vi "Actor Core.vi"(8 "error in":errorcluster, 11 "TestQList in":refnum<class "TestQList.lvclass">) -> (0 "error out":errorcluster, 3 "Actor out":refnum<class "Actor.lvclass">)   [LabVIEW 2019, in "TestQList.lvclass"]
doc: "(<B>Filename</B>: Actor Framework.lvlib:Actor.lvclass:Actor Core.vi)\n\nReceives messages to the actor, reacts to them, and initiates any error handling that may shut the actor down.\n\nDescendant classes may override this VI to append parallel tasks for the actor to complete while it handles messages. Overrides use the Call Parent Method node."
uses:
  TestQList.lvclass
  C:/Program Files/National Instruments/LabVIEW 2019/vi.lib/ActorFramework/Actor/Actor.lvclass
  <vilib>/ActorFramework/Actor/Actor.lvclass
  Queued Listbox.xctl
  <vilib>/ActorFramework/Actor/Actor.lvclass/Actor.ctl
  <vilib>/ActorFramework/Message Enqueuer/Message Enqueuer.lvclass/Message Enqueuer.ctl
  <vilib>/ActorFramework/Message Enqueuer/Init from Existing Queue.vi
  <vilib>/ActorFramework/Message Enqueuer/Enqueue.vi
  <vilib>/ActorFramework/Stop Msg/Stop Msg.lvclass
  C:/Program Files/National Instruments/LabVIEW 2019/vi.lib/ActorFramework/Message/Message.lvclass
  <vilib>/ActorFramework/Message Priority Queue/Priority Enqueue.vi
  <vilib>/ActorFramework/Message Enqueuer/Message Enqueuer.lvclass
panel:
  in  "Stop Button":bool
  in  "Queued Listbox":string[](xcontrol)
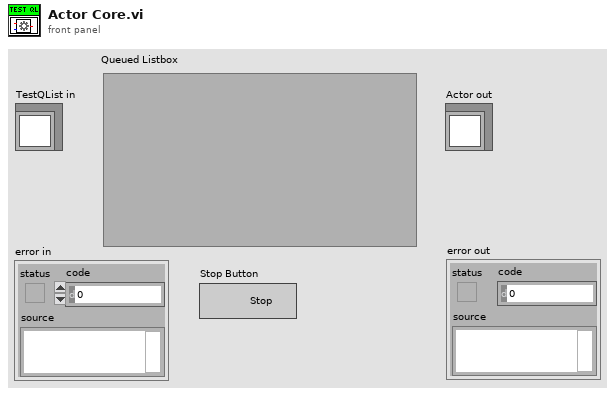
[diagram p1: front panel]
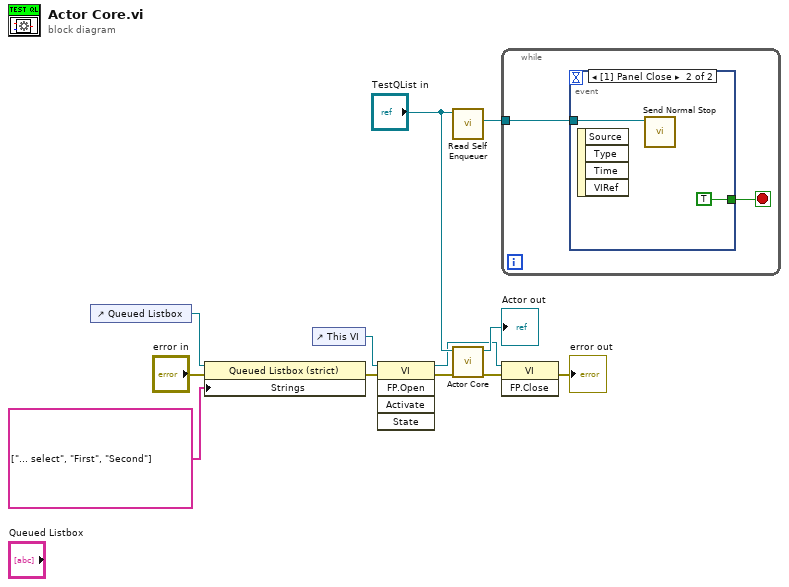
[diagram p0: block diagram]
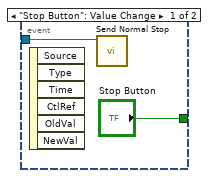
[diagram p2: hidden frame]
diagram:
  n1 = control-ref of="Queued Listbox"() -> (w4:refnum<vi>)
  n2 = property class="Queued Listbox (strict)"(reference=w4, error in="error in", "Strings"=string[] ["... select", "First", "Second"]) -> (error out=w2:errorcluster)  [unwired: 1 out]
  n3 = control-ref of="This VI"() -> (w9:refnum<vi>)
  n4 = invoke class="VI" method="FP.Open"(reference=w9, error in=w2) -> (reference out=w6:refnum<vi>, error out=w8:errorcluster)  [unwired: 3 in, 3 out]
  n5 = call <vilib>:"Read Self Enqueuer.vi"("Actor"="TestQList in") -> ("Self Enqueuer"=w10:refnum<class "Message Enqueuer.lvclass">)  [unwired: 10 in]
  n6 = call-parent "Actor Core.vi"("error in"=w8, "Actor in"="TestQList in") -> ("error out"=w7:errorcluster, "Actor out"=→"Actor out":refnum<class "Actor.lvclass">)  [unwired: 8 in]
  n7 = while {
    tunnel: w10 -> [w14]
    stop <- w13 stop-if-true
    n8 = event shown="[1] Panel Close" {
      selector: _ -> [_ _]
      dyn-events: _ -> [_ _]
      timeout: _ -> [_ _]
      tunnel: w14 -> [w16 w18]
      tunnel: ["Stop Button" TRUE ("Stop Button")] -> w13
      event "Stop Button": Value Change {
        n9 = event-data() -> ()  [unwired: 1 in, 6 out]
        n10 = call <vilib>:"Send Normal Stop.vi"("Message Enqueuer"=w16) -> ()  [unwired: 10 in, 1 out]
      }
      event Panel Close {
        n11 = event-data() -> ()  [unwired: 1 in, 4 out]
        n12 = call <vilib>:"Send Normal Stop.vi"("Message Enqueuer"=w18) -> ()  [unwired: 10 in, 1 out]
      }
    }
  }
  n13 = invoke class="VI" method="FP.Close"(reference=w6, error in=w7) -> (error out=→"error out":errorcluster)  [unwired: 1 in, 2 out]
